vi "Barcode user prompt.vi"() -> (2 "BARCODE":string)   [LabVIEW 2021]
uses:
  <vilib>/regexp/Match Regular Expression.xnode
panel:
  in  "Ok":bool
  in  "Input Barcode":string
  # "Please scan barcode or type its corresponding value in below field & press OK"
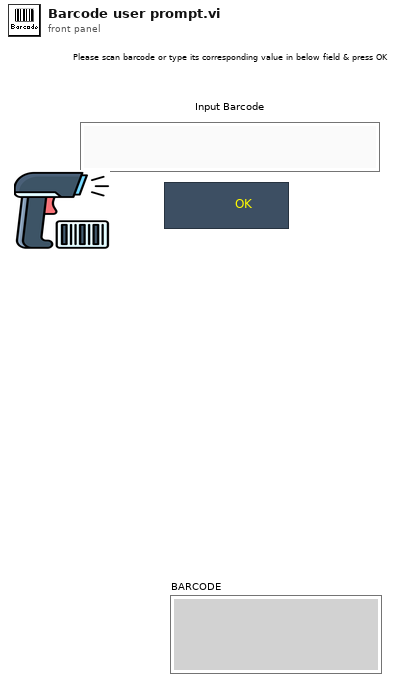
[diagram p1: front panel]
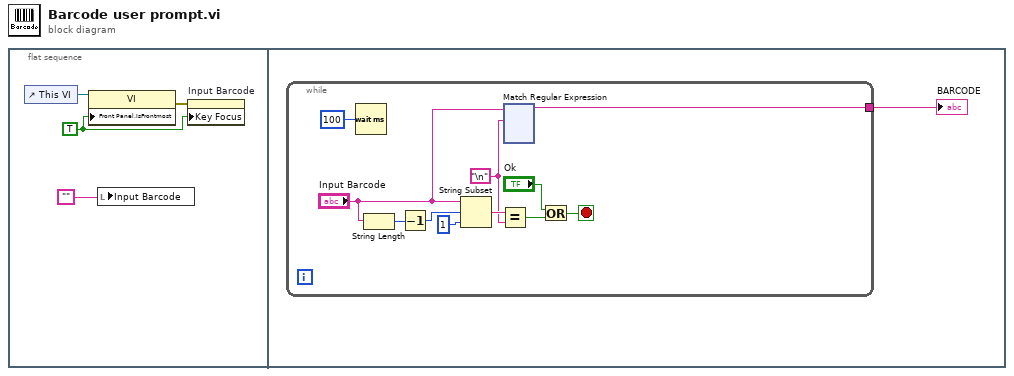
[diagram p0: block diagram]
diagram:
  n1 = flat-sequence {
    frame #0 {
      w2 = TRUE ("Front Panel Window:Is Frontmost")
      n2 = control-ref of="This VI"() -> (w4:refnum<vi>)
      n3 = property class="VI"(reference=w4, "Front Panel.IsFrontmost"=w2) -> (error out=w3:errorcluster)  [unwired: 1 in, 1 out]
      n4 = local write "Input Barcode"("") -> ()
      n5 = property on="Input Barcode" class="Str"(error in=w3, "Key Focus"=w2) -> ()  [unwired: 1 in, 2 out]
    }
    frame #1 {
      n6 = while {
        tunnel: [w7] -> w5
        stop <- w10 stop-if-true
        w8 = "\n"
        n7 = Wait (ms)(milliseconds to wait=u32 100) -> ()  [unwired: 1 out]
        n8 = String Length(string="Input Barcode") -> (length=w15:i32)
        n9 = Decrement(x=w15) -> (x-1=w14:i32)
        n10 = String Subset(string="Input Barcode", offset (0)=w14, length (rest)=1 ("length (rest)")) -> (substring=w11:string)
        n11 = Equal?(x=w11, y=w8) -> (x = y?=w6:bool)
        n12 = xnode "Match Regular Expression"("input string"="Input Barcode", "regular expression"=w8) -> ("before match"=w7:string)  [unwired: 4 in, 4 out]
        n13 = Or(x="Ok", y=w6) -> (x .or. y?=w10:bool)
      }
      "BARCODE" <- w5
    }
  }
